vi "Full Force Test 2.vi"(8 "error in (no error)":errorcluster, 10 "Model in":refnum<class "Model.lvclass">, 11 "Test Actuator State in":refnum<class "Test Actuator State.lvclass">) -> (0 "error out":errorcluster, 2 "Model out":refnum<class "Model.lvclass">, 3 "Test Actuator State out":refnum<class "Test Actuator State.lvclass">)   [LabVIEW 2016, in "Test Actuator State.lvclass"]
uses:
  Test Actuator State.lvclass
  Model/Model/Model.lvclass
  Typedefs/ActuatorSetPoints.ctl
  Typedefs/FAMT Typedefs.lvlib
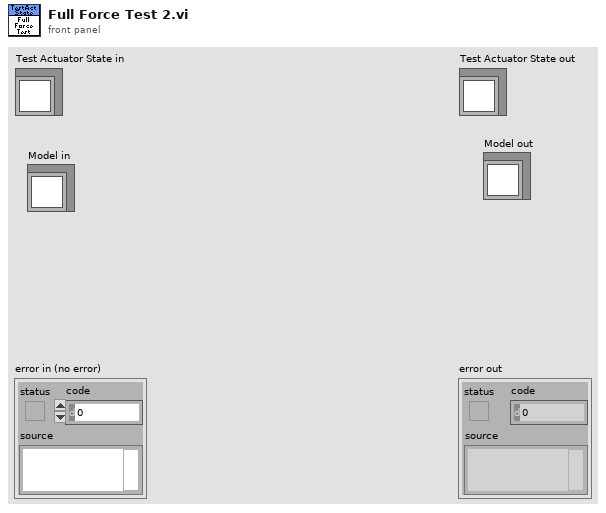
[diagram p1: front panel]
types:
  T1 = typedef "FAMT Typedefs.lvlib/FullForceScanSettings.ctl" = cluster{"Force Tolerance (N)":dbl, "DAA Force Set Points":T2[], "Process Time (s)":dbl, "Sample Time (s)":dbl, "Max Moment (NM)":dbl, "SAA Force Set Points":T2[]}
  T2 = typedef "FAMT Typedefs.lvlib/ForcePair.ctl" = cluster{"Axial Force":dbl, "Lateral Force":dbl}
  T3 = typedef "FAMT Typedefs.lvlib/ActuatorSetPoints.ctl" = cluster{"Axial Force":dbl, "Lateral Force":dbl, "FC1 Force":dbl, "FC2 Force":dbl}
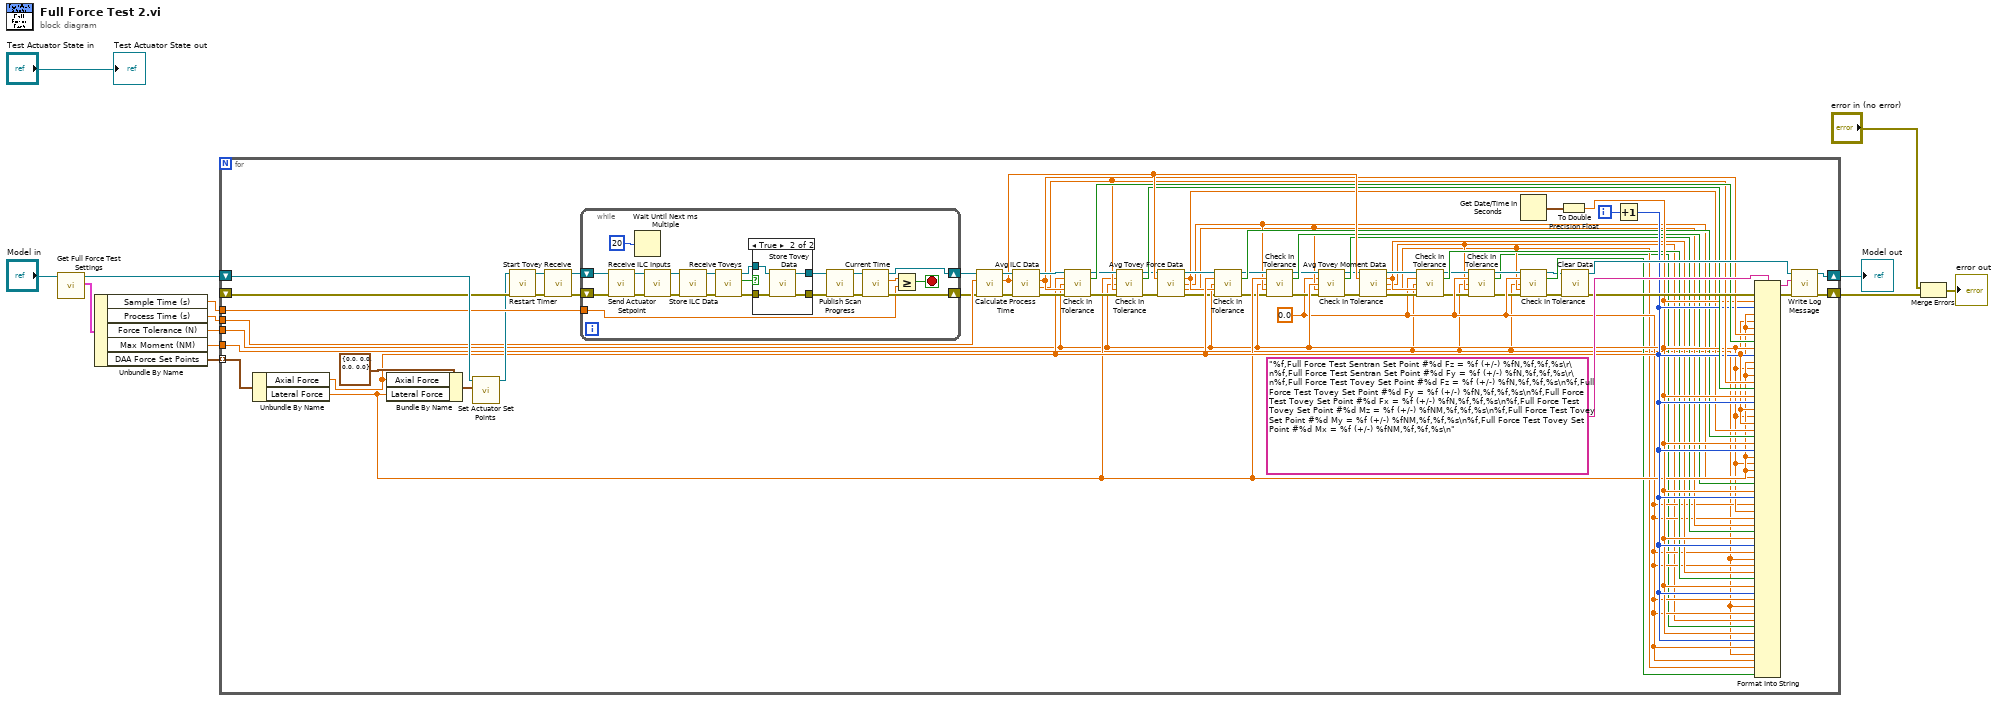
[diagram p0: block diagram]
diagram:
  n1 = call "Get Full Force Test Settings.vi"("Model in"="Model in") -> ("Full Force Test Settings"=w2:T1, "Model out"=w12:refnum<class "Model.lvclass">)  [unwired: 9 in]
  n2 = Unbundle By Name(w2) -> ("Sample Time (s)"=w11:dbl, "Process Time (s)"=w10:dbl, "Force Tolerance (N)"=w9:dbl, "Max Moment (NM)"=w4:dbl, "DAA Force Set Points"=w1:T2[])
  n3 = for {
    tunnel: w1 -> [w69] mode=indexing
    shift-right: [w79] -> w6
    shift-left: w12 -> [w83]
    tunnel: w11 -> [w82]
    tunnel: w10 -> [w64]
    tunnel: w9 -> [w37]
    shift-right: [w65] -> w5
    shift-left: _ -> [w81]
    tunnel: w4 -> [w14]
    i -> [w76]
    w23 = 0.0
    n4 = Unbundle By Name(w69) -> ("Axial Force"=w45:dbl, "Lateral Force"=w41:dbl)
    n5 = Bundle By Name(cluster=T3 {"Axial Force"=0.0, "Lateral Force"=0.0, "FC1 Force"=0.0, "FC2 Force"=0.0} ("Actuator Set Points"), "Axial Force"=w45, "Lateral Force"=w41) -> (w70:T3)
    n6 = call "Set Actuator Set Points.vi"("Actuator Set Points"=w70, "Model in"=w83) -> ("Model out"=w71:refnum<class "Model.lvclass">)  [unwired: 9 in]
    n7 = call "Restart Timer.vi"("error in (no error)"=w81, "Model in"=w71) -> ("error out"=w74:errorcluster, "Model out"=w75:refnum<class "Model.lvclass">)  [unwired: 8 in]
    n8 = call "Start Tovey Receive.vi"("error in (no error)"=w74, "Model in"=w75) -> ("error out"=w72:errorcluster, "Model out"=w73:refnum<class "Model.lvclass">)  [unwired: 8 in]
    n9 = while {
      shift-right: [w98] -> w63
      shift-left: w73 -> [w104]
      shift-right: [w97] -> w61
      shift-left: w72 -> [w101]
      tunnel: w82 -> [w95]
      stop <- w94 stop-if-true
      n10 = call "Send Actuator Setpoint.vi"("error in (no error)"=w101, "Model in"=w104) -> ("error out"=w100:errorcluster, "Model out"=w103:refnum<class "Model.lvclass">)  [unwired: 8 in]
      n11 = Wait Until Next ms Multiple(millisecond multiple=u32 20) -> ()  [unwired: 1 out]
      n12 = call "Receive ILC Inputs.vi"("error in (no error)"=w100, "Model in"=w103) -> ("error out"=w99:errorcluster, "Model out"=w102:refnum<class "Model.lvclass">)  [unwired: 8 in]
      n13 = call "Store ILC Data.vi"("error in (no error)"=w99, "Model in"=w102) -> ("error out"=w92:errorcluster, "Model out"=w93:refnum<class "Model.lvclass">)  [unwired: 8 in]
      n14 = call "Receive Toveys.vi"("error in (no error)"=w92, "Model in"=w93) -> ("error out"=w90:errorcluster, "Data Received"=w89:bool, "Model out"=w91:refnum<class "Model.lvclass">)  [unwired: 7 in]
      n15 = case shown="True" w89 {
        tunnel: w91 -> [w107 w111]
        tunnel: w90 -> [w106 w110]
        tunnel: [w106 w109] -> w85
        tunnel: [w107 w108] -> w88
        frame False {
        }
        frame True {
          n16 = call "Store Tovey Data.vi"("error in (no error)"=w110, "Model in"=w111) -> ("error out"=w109:errorcluster, "Model out"=w108:refnum<class "Model.lvclass">)  [unwired: 8 in]
        }
      }
      n17 = call "Publish Scan Progress.vi"("error in (no error)"=w85, "Model in"=w88) -> ("error out"=w86:errorcluster, "Model out"=w87:refnum<class "Model.lvclass">)  [unwired: 8 in]
      n18 = call "Current Time.vi"("error in (no error)"=w86, "Model in"=w87) -> ("error out"=w97:errorcluster, "Time"=w96:dbl, "Model out"=w98:refnum<class "Model.lvclass">)  [unwired: 7 in]
      n19 = Greater Or Equal?(x=w96, y=w95) -> (x >= y?=w94:bool)
    }
    n20 = call "Calculate Process Time.vi"("error in (no error)"=w61, "Seconds"=w64, "Model in"=w63) -> ("error out"=w60:errorcluster, "Time"=w59:dbl, "Model out"=w62:refnum<class "Model.lvclass">)  [unwired: 6 in]
    n21 = call "Avg ILC Data.vi"("error in (no error)"=w60, "After This Time"=w59, "Model in"=w62) -> ("error out"=w52:errorcluster, "Fy"=w54:dbl, "Fz"=w57:dbl, "Model out"=w58:refnum<class "Model.lvclass">)  [unwired: 5 in]
    n22 = call "Check In Tolerance.vi"("Model in"=w58, "Expected"=w45, "Tolerance"=w37, "Actual"=w57, "error in (no error)"=w52) -> ("Model out"=w55:refnum<class "Model.lvclass">, "Pass"=w56:bool, "error out"=w51:errorcluster)  [unwired: 8 in]
    n23 = call "Check In Tolerance.vi"("Model in"=w55, "Expected"=w41, "Tolerance"=w37, "Actual"=w54, "error in (no error)"=w51) -> ("Model out"=w49:refnum<class "Model.lvclass">, "Pass"=w53:bool, "error out"=w50:errorcluster)  [unwired: 8 in]
    n24 = call "Avg Tovey Force Data.vi"("Model in"=w49, "After This Time"=w59, "error in (no error)"=w50) -> ("Model out"=w46:refnum<class "Model.lvclass">, "Fz"=w43:dbl, "Fy"=w39:dbl, "Fx"=w27:dbl, "error out"=w34:errorcluster)  [unwired: 8 in]
    n25 = call "Check In Tolerance.vi"("Model in"=w46, "Expected"=w45, "Tolerance"=w37, "Actual"=w43, "error in (no error)"=w34) -> ("Model out"=w42:refnum<class "Model.lvclass">, "Pass"=w44:bool, "error out"=w33:errorcluster)  [unwired: 8 in]
    n26 = call "Check In Tolerance.vi"("Model in"=w42, "Expected"=w41, "Tolerance"=w37, "Actual"=w39, "error in (no error)"=w33) -> ("Model out"=w38:refnum<class "Model.lvclass">, "Pass"=w40:bool, "error out"=w32:errorcluster)  [unwired: 8 in]
    n27 = call "Check In Tolerance.vi"("Model in"=w38, "Expected"=w23, "Tolerance"=w37, "Actual"=w27, "error in (no error)"=w32) -> ("Model out"=w30:refnum<class "Model.lvclass">, "Pass"=w36:bool, "error out"=w31:errorcluster)  [unwired: 8 in]
    n28 = call "Avg Tovey Moment Data.vi"("Model in"=w30, "After This Time"=w59, "error in (no error)"=w31) -> ("Model out"=w29:refnum<class "Model.lvclass">, "Mz"=w26:dbl, "My"=w22:dbl, "Mx"=w21:dbl, "error out"=w28:errorcluster)  [unwired: 8 in]
    n29 = call "Check In Tolerance.vi"("Model in"=w29, "Expected"=w23, "Tolerance"=w14, "Actual"=w26, "error in (no error)"=w28) -> ("Model out"=w25:refnum<class "Model.lvclass">, "Pass"=w35:bool, "error out"=w17:errorcluster)  [unwired: 8 in]
    n30 = call "Check In Tolerance.vi"("Model in"=w25, "Expected"=w23, "Tolerance"=w14, "Actual"=w22, "error in (no error)"=w17) -> ("Model out"=w24:refnum<class "Model.lvclass">, "Pass"=w20:bool, "error out"=w16:errorcluster)  [unwired: 8 in]
    n31 = Get Date/Time In Seconds() -> (seconds since 1Jan1904=w77:timestamp)
    n32 = call "Check In Tolerance.vi"("Model in"=w24, "Expected"=w23, "Tolerance"=w14, "Actual"=w21, "error in (no error)"=w16) -> ("Model out"=w18:refnum<class "Model.lvclass">, "Pass"=w19:bool, "error out"=w15:errorcluster)  [unwired: 8 in]
    n33 = To Double Precision Float(number=w77) -> (double precision float=w47:dbl)
    n34 = call "Clear Data.vi"("error in (no error)"=w15, "Model in"=w18) -> ("error out"=w67:errorcluster, "Model out"=w80:refnum<class "Model.lvclass">)  [unwired: 8 in]
    n35 = Increment(x=w76) -> (x+1=w48:i32)
    n36 = Format Into String(format string="%f,Full Force Test Sentran Set Point #%d Fz = %f (+/-) %fN,%f,%f,%s\r\n%f,Full Force Test Sentran Set Point #%d Fy = %f (+/-) %fN,%f,%f,%s\r\n%f,Full Force Test Tovey Set Point #%d Fz = %f (+/-) %fN,%f,%f,%s\n%f,Full Force Test Tovey Set Point #%d Fy = %f (+/-) %fN,%f,%f,%s\n%f,Full Force Test Tovey Set Point #%d Fx = %f (+/-) %fN,%f,%f,%s\n%f,Full Force Test Tovey Set Point #%d Mz = %f (+/-) %fNM,%f,%f,%s\n%f,Full Force Test Tovey Set Point #%d My = %f (+/-) %fNM,%f,%f,%s\n%f,Full Force Test Tovey Set Point #%d Mx = %f (+/-) %fNM,%f,%f,%s\n", error in=w67, w47, w48, w45, w37, w45, w57, w56, w47, w48, w41, w37, w41, w54, w53, w47, w48, w45, w37, w45, w43, w44, w47, w48, w41, w37, w41, w39, w40, w47, w48, w23, w37, w23, w27, w36, w47, w48, w23, w14, w23, w26, w35, w47, w48, w23, w14, w23, w22, w20, w47, w48, w23, w14, w23, w21, w19) -> (resulting string=w68:string, error out=w66:errorcluster)  [unwired: 1 in]
    n37 = call "Write Log Message.vi"("error in (no error)"=w66, "Message"=w68, "Model in"=w80) -> ("error out"=w65:errorcluster, "Model out"=w79:refnum<class "Model.lvclass">)  [unwired: 7 in]
  }
  "Model out" <- w6
  n38 = Merge Errors("error in (no error)", w5) -> (→"error out":errorcluster)
  "Test Actuator State out" <- "Test Actuator State in"
